vi "Get Package Version.vi"(8 "error in (no error)":errorcluster, 10 "package name":string, 11 "NI Package Builder solution (.pbs)":path) -> (0 "error out":errorcluster, 1 "version":string, 2 "package name out":string, 3 "NI Package Builder solution out":path)   [LabVIEW 2017, in "NIPB Solution API.lvlib"]
doc: "Gets the version of the specified package in the specified NI Package Builder solution (.pbs).\n\nIf the <b>package name</b> input is unwired, this VI will perform this operation on the first package in the NI Package Builder solution and output the corresponding package name in the <b>package name out</b> output."
uses:
  NIPB Solution API.lvlib
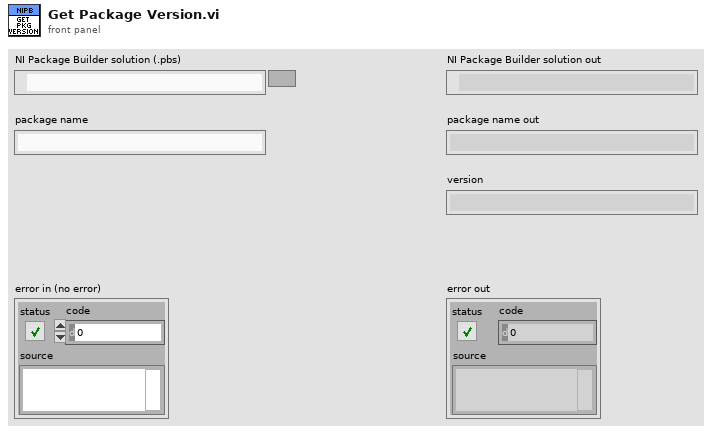
[diagram p1: front panel]
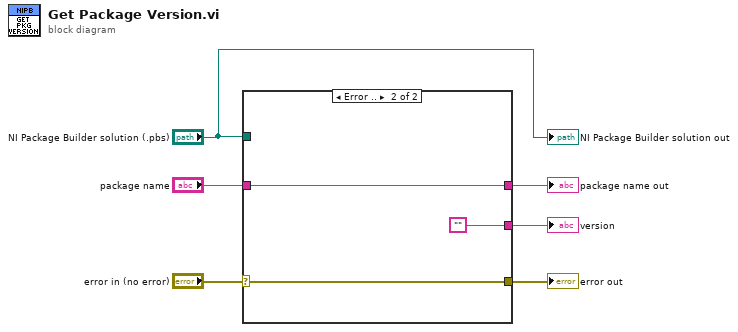
[diagram p0: block diagram]
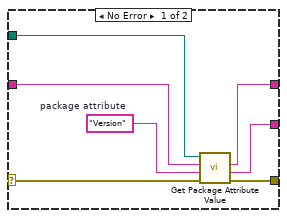
[diagram p2: hidden frame]
diagram:
  n1 = case shown="Error .." "error in (no error)" {
    selector: "error in (no error)" -> [w13 w16]
    tunnel: [w12 w16] -> w5
    tunnel: "NI Package Builder solution (.pbs)" -> [w10 _]
    tunnel: "package name" -> [w11 w14]
    tunnel: [w8 ""] -> w3
    tunnel: [w7 w14] -> w1
    frame No Error {
      w9 = "Version"  # package attribute
      n2 = call "Get Package Attribute Value.vi"("error in (no error)"=w13, "package attribute"=w9, "package name"=w11, "NI Package Builder solution (.pbs)"=w10) -> ("error out"=w12:errorcluster, "Value"=w8:string, "package name out"=w7:string)  [unwired: 4 in, 1 out]
    }
    frame Error {
    }
  }
  "version" <- w3
  "error out" <- w5
  "package name out" <- w1
  "NI Package Builder solution out" <- "NI Package Builder solution (.pbs)"
